vi "Multicard III_Hardware_Module.vi"(5 "Multicard (T:Enable)":bool=TRUE, 6 "Timeout(s)":dbl=5.0, 7 "Command":T1, 8 "error in (no error)":errorcluster, 10 "Input Value":dbl, 11 "VISA resource name":refnum<visa-resource-name>="COM4") -> (0 "error out":errorcluster, 1 "Timeout":bool, 2 "Output Value":dbl=5.0, 3 "String":string)   [LabVIEW 2013]
uses:
  Multicard III_Hardware_Module Control.ctl
  <vilib>/Instr/_visa.llb/VISA Configure Serial Port (Instr).vi
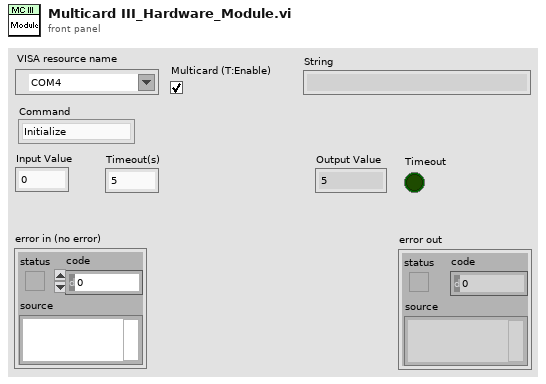
[diagram p1: front panel]
types:
  T1 = typedef "Multicard III_Hardware_Module Control.ctl" = enum16{"Initialize", "Cero", "Span", "Read ugr", "Read mgr", "Read A/D", "Read T", "Number readings", "Thermocouple type", "Status", "Shutdown"}
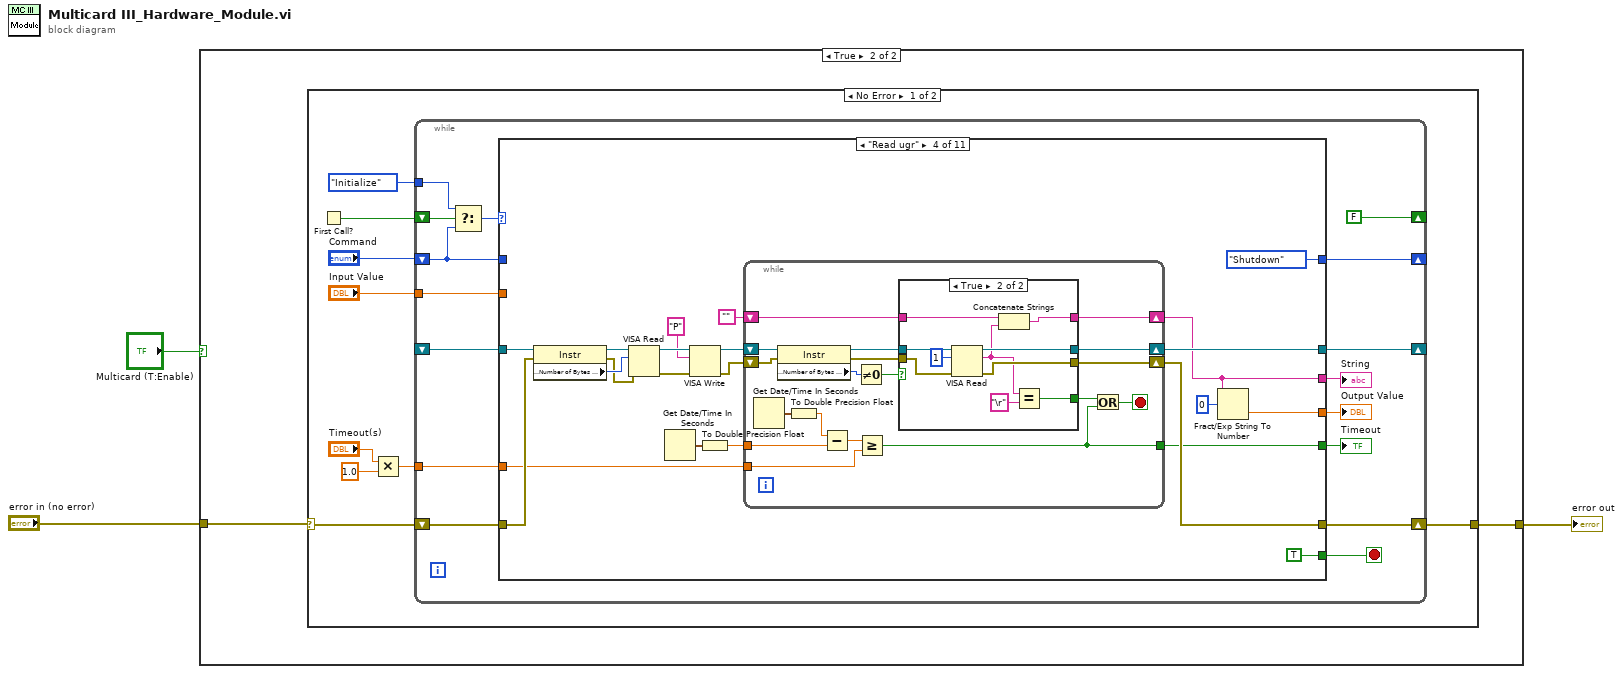
[diagram p0: block diagram]
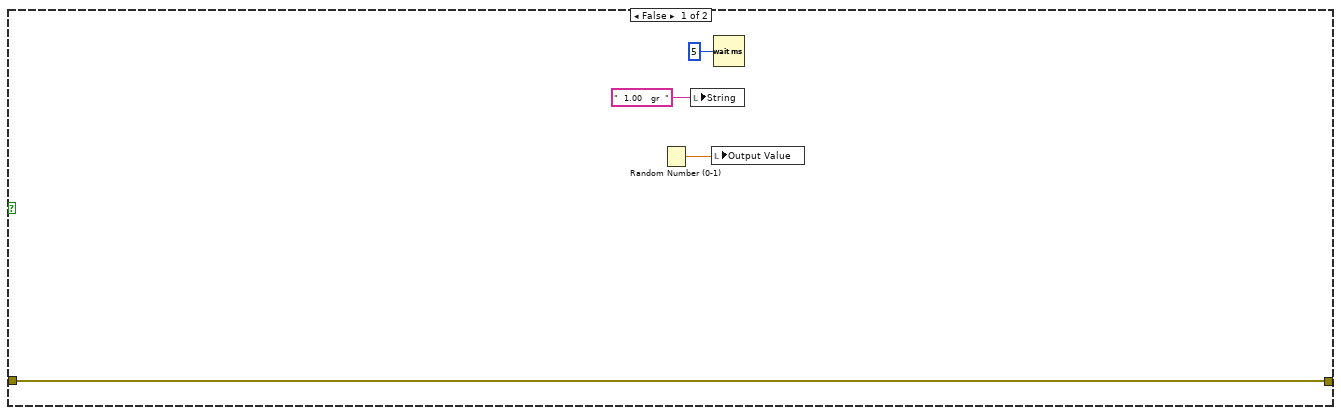
[diagram p2: hidden frame]
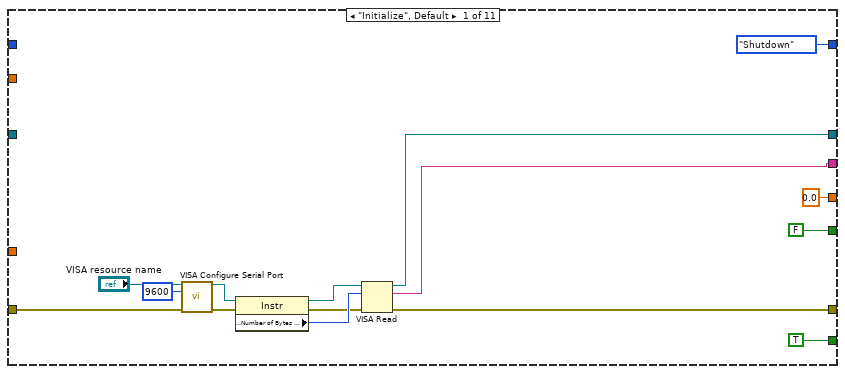
[diagram p3: hidden frame]
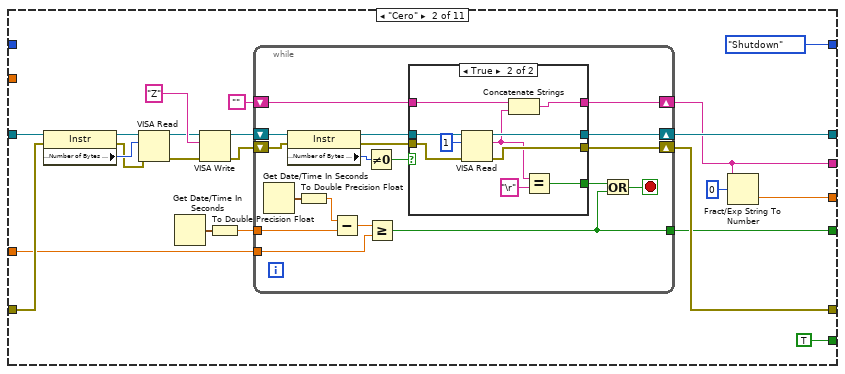
[diagram p4: hidden frame]
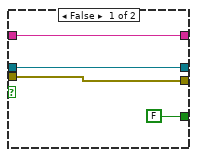
[diagram p5: hidden frame]
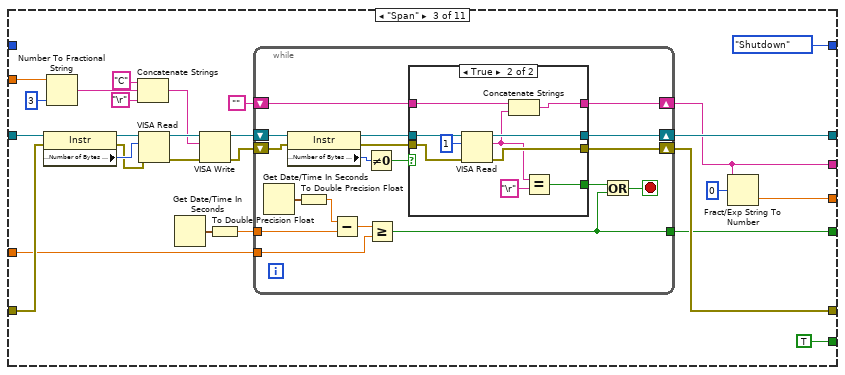
[diagram p6: hidden frame]
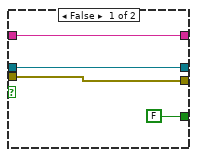
[diagram p7: hidden frame]
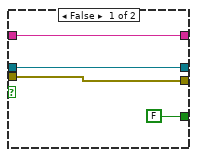
[diagram p8: hidden frame]
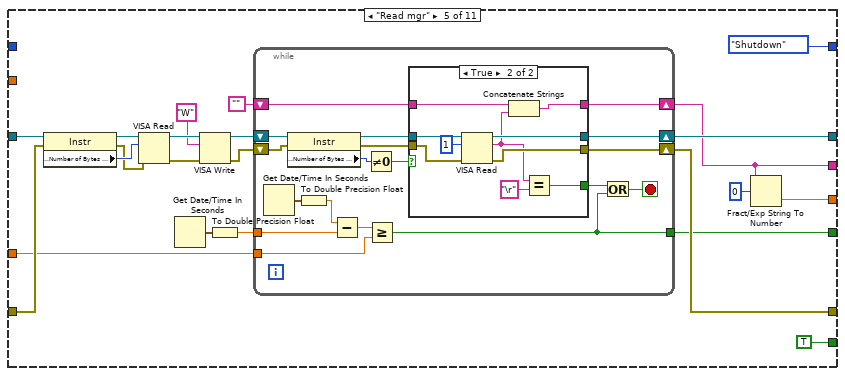
[diagram p9: hidden frame]
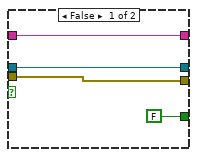
[diagram p10: hidden frame]
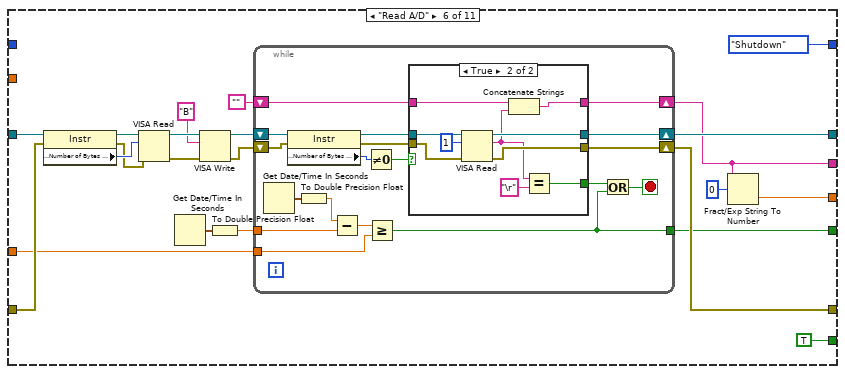
[diagram p11: hidden frame]
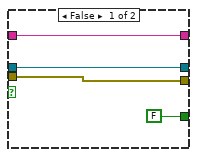
[diagram p12: hidden frame]
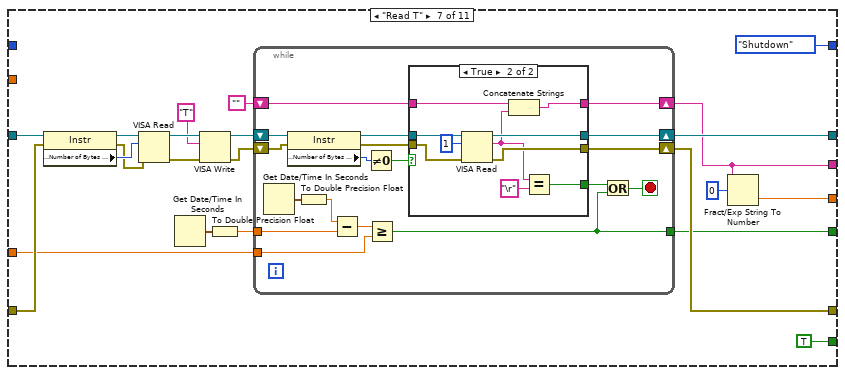
[diagram p13: hidden frame]
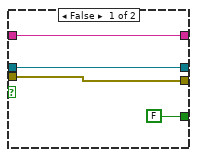
[diagram p14: hidden frame]
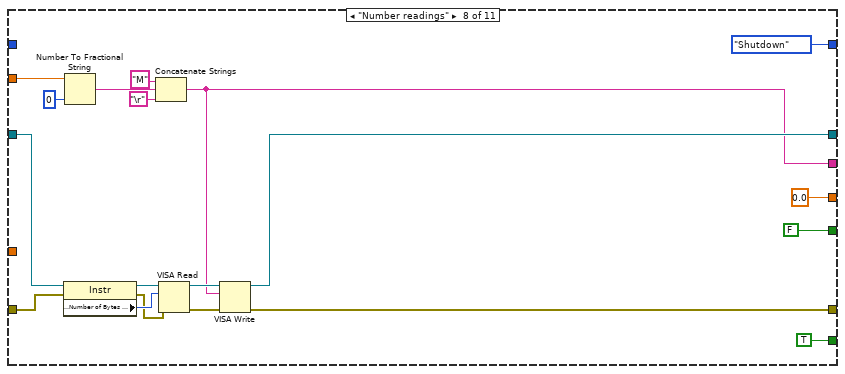
[diagram p15: hidden frame]
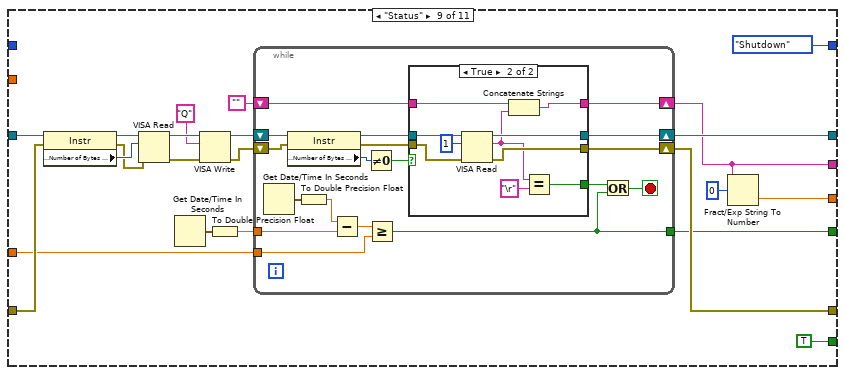
[diagram p16: hidden frame]
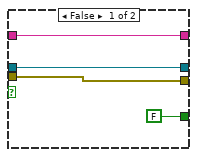
[diagram p17: hidden frame]
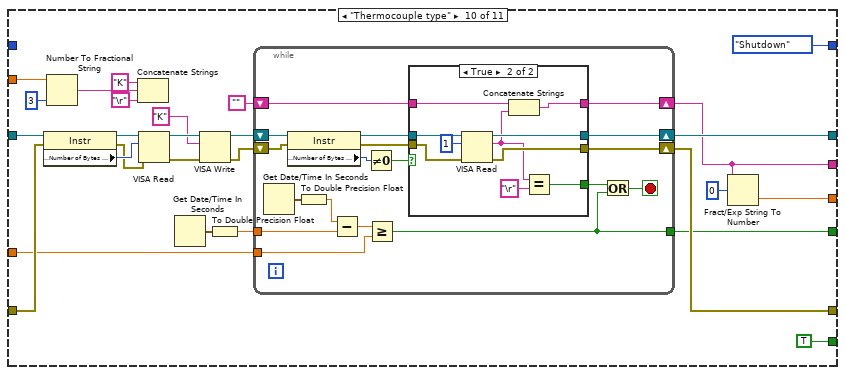
[diagram p18: hidden frame]
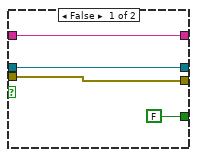
[diagram p19: hidden frame]
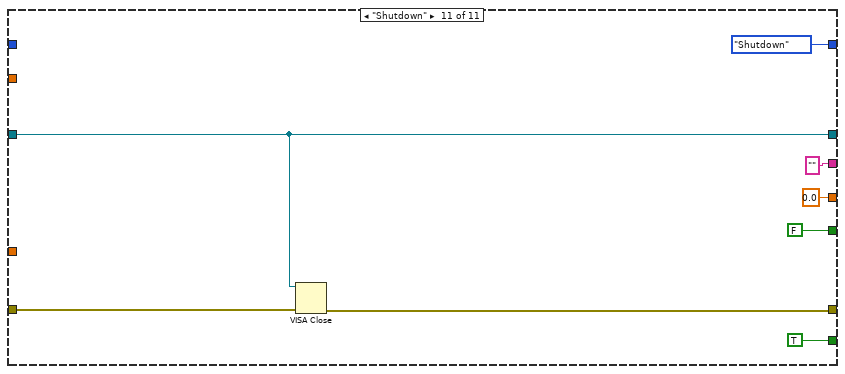
[diagram p20: hidden frame]
diagram:
  n1 = case shown="True" "Multicard (T:Enable)" {
    tunnel: "error in (no error)" -> [w7 w9]
    tunnel: [w7 w8] -> w2
    frame False {
      n2 = Random Number (0-1)() -> (number: 0 to 1=w5:dbl)
      n3 = local write "String"("  1.00   gr  " ("String")) -> ()
      n4 = local write "Output Value"(w5) -> ()
      n5 = Wait (ms)(milliseconds to wait=u32 5) -> ()  [unwired: 1 out]
    }
    frame True {
      n6 = case shown="No Error" w9 {
        selector: w9 -> [w16 w519]
        tunnel: [w15 w519] -> w8
        frame No Error {
          n7 = First Call?() -> (First Call?: T/F=w18:bool)
          n8 = Multiply(x="Timeout(s)", y=1.0) -> (x*y=w11:dbl)
          n9 = while {
            shift-right: [w26] -> _
            shift-left: "Command" -> [w27]
            shift-right: [w29] -> w15
            shift-left: w16 -> [w30]
            shift-right: [FALSE ("First Call?: T/F")] -> _
            shift-left: w18 -> [w34]
            tunnel: Multicard_III_Hardware_Module_Control."Initialize" ("t") -> [w33]
            shift-right: [w24] -> _
            shift-left: _ -> [w25]
            tunnel: w11 -> [w22]
            tunnel: "Input Value" -> [w19]
            stop <- w31 stop-if-true
            n10 = Select(t=w33, s=w34, f=w27) -> (s? t:f=w32:T1)
            n11 = case shown="\"Read ugr\"" w32 {
              tunnel: [TRUE TRUE TRUE TRUE TRUE TRUE TRUE TRUE TRUE TRUE TRUE] -> w31
              tunnel: w30 -> [w46 w58 w118 w172 w226 w280 w334 w390 w407 w466 w518]
              tunnel: [w39 w59 w119 w173 w227 w281 w335 w379 w408 w467 w517] -> w29
              tunnel: w27 -> [_ _ _ _ _ _ _ _ _ _ _]
              tunnel: [Multicard_III_Hardware_Module_Control."Shutdown" ("t") Multicard_III_Hardware_Module_Control."Shutdown" ("t") Multicard_III_Hardware_Module_Control."Shutdown" ("t") Multicard_III_Hardware_Module_Control."Shutdown" ("t") Multicard_III_Hardware_Module_Control."Shutdown" ("t") Multicard_III_Hardware_Module_Control."Shutdown" ("t") Multicard_III_Hardware_Module_Control."Shutdown" ("t") Multicard_III_Hardware_Module_Control."Shutdown" ("t") Multicard_III_Hardware_Module_Control."Shutdown" ("t") Multicard_III_Hardware_Module_Control."Shutdown" ("t") Multicard_III_Hardware_Module_Control."Shutdown" ("t")] -> w26
              tunnel: w25 -> [_ w57 w117 w171 w225 w279 w333 w389 w406 w465 w516]
              tunnel: [w38 w55 w115 w169 w223 w277 w331 w383 w404 w463 w516] -> w24
              tunnel: [w36 w52 w112 w166 w220 w274 w328 w382 w401 w460 ""] -> w23
              tunnel: w22 -> [_ w56 w116 w170 w224 w278 w332 _ w405 w464 _]
              tunnel: [FALSE w53 w113 w167 w221 w275 w329 FALSE w402 w461 FALSE] -> w21
              tunnel: [0.0 w51 w111 w165 w219 w273 w327 0.0 w400 w459 0.0] -> w20
              tunnel: w19 -> [_ _ w106 _ _ _ _ w384 _ w456 _]
              frame "Initialize", Default {
                n12 = call-poly "VISA Configure Serial Port"("VISA resource name"="VISA resource name", "baud rate (9600)"=u32 9600, "error in (no error)"=w46) -> ("VISA resource name out"=w41:refnum<visa-resource-name>, "error out"=w40:errorcluster)  [unwired: 11 in]
                n13 = property class="Instr"(reference=w41, error in=w40) -> (reference out=w42:refnum<visa-resource-name>, error out=w43:errorcluster, "Serial Settings:Number of Bytes at Serial Port"=w44:u32)
                n14 = VISA Read(VISA resource name=w42, byte count=w44, error in (no error)=w43) -> (VISA resource name out=w38:refnum<visa-resource-name>, read buffer=w36:string, error out=w39:errorcluster)  [unwired: 1 out]
              }
              frame "Cero" {
                n15 = property class="Instr"(reference=w57, error in=w58) -> (reference out=w66:refnum<visa-resource-name>, error out=w67:errorcluster, "Serial Settings:Number of Bytes at Serial Port"=w68:u32)
                n16 = VISA Read(VISA resource name=w66, byte count=w68, error in (no error)=w67) -> (VISA resource name out=w65:refnum<visa-resource-name>, error out=w64:errorcluster)  [unwired: 2 out]
                n17 = Get Date/Time In Seconds() -> (seconds since 1Jan1904=w63:timestamp)
                n18 = VISA Write(VISA resource name=w65, write buffer="Z" ("Mide"), error in (no error)=w64) -> (VISA resource name out=w61:refnum<visa-resource-name>, error out=w60:errorcluster)  [unwired: 1 out]
                n19 = To Double Precision Float(number=w63) -> (double precision float=w62:dbl)
                n20 = while {
                  tunnel: w62 -> [w86]
                  shift-right: [w82] -> w55
                  shift-left: w61 -> [w80]
                  shift-right: [w81] -> w59
                  shift-left: w60 -> [w79]
                  tunnel: w56 -> [w84]
                  tunnel: [w83] -> w53
                  shift-right: [w73] -> w52
                  shift-left: "" -> [w74]
                  stop <- w89 stop-if-true
                  n21 = Get Date/Time In Seconds() -> (seconds since 1Jan1904=w88:timestamp)
                  n22 = property class="Instr"(reference=w80, error in=w79) -> (reference out=w77:refnum<visa-resource-name>, error out=w78:errorcluster, "Serial Settings:Number of Bytes at Serial Port"=w76:u32)
                  n23 = To Double Precision Float(number=w88) -> (double precision float=w87:dbl)
                  n24 = Subtract(x=w87, y=w86) -> (x-y=w85:dbl)
                  n25 = Not Equal To 0?(x=w76) -> (x != 0?=w75:bool)
                  n26 = Greater Or Equal?(x=w85, y=w84) -> (x >= y?=w83:bool)
                  n27 = case shown="True" w75 {
                    tunnel: [w93 w103] -> w82
                    tunnel: [w92 w102] -> w81
                    tunnel: w78 -> [w92 w101]
                    tunnel: w77 -> [w93 w100]
                    tunnel: w74 -> [w91 w99]
                    tunnel: [w91 w98] -> w73
                    tunnel: [FALSE w94] -> w72
                    frame False {
                    }
                    frame True {
                      n28 = VISA Read(VISA resource name=w100, byte count=u32 1, error in (no error)=w101) -> (VISA resource name out=w103:refnum<visa-resource-name>, read buffer=w96:string, error out=w102:errorcluster)  [unwired: 1 out]
                      n29 = Concatenate Strings(w99, w96) -> (w98:string)
                      n30 = Equal?(x=w96, y="\r" ("Mide")) -> (x = y?=w94:bool)
                    }
                  }
                  n31 = Or(x=w72, y=w83) -> (x .or. y?=w89:bool)
                }
                n32 = Fract/Exp String To Number(string=w52, offset=0) -> (number=w51:dbl)  [unwired: 2 in, 1 out]
              }
              frame "Span" {
                n33 = property class="Instr"(reference=w117, error in=w118) -> (reference out=w126:refnum<visa-resource-name>, error out=w127:errorcluster, "Serial Settings:Number of Bytes at Serial Port"=w128:u32)
                n34 = Number To Fractional String(number=w106, precision (6)=i16 3) -> (F-format string=w104:string)  [unwired: 2 in]
                n35 = Concatenate Strings("C" ("Mide"), w104, "\r") -> (w107:string)
                n36 = VISA Read(VISA resource name=w126, byte count=w128, error in (no error)=w127) -> (VISA resource name out=w125:refnum<visa-resource-name>, error out=w124:errorcluster)  [unwired: 2 out]
                n37 = Get Date/Time In Seconds() -> (seconds since 1Jan1904=w123:timestamp)
                n38 = VISA Write(VISA resource name=w125, write buffer=w107, error in (no error)=w124) -> (VISA resource name out=w121:refnum<visa-resource-name>, error out=w120:errorcluster)  [unwired: 1 out]
                n39 = To Double Precision Float(number=w123) -> (double precision float=w122:dbl)
                n40 = while {
                  tunnel: w122 -> [w145]
                  shift-right: [w141] -> w115
                  shift-left: w121 -> [w139]
                  shift-right: [w140] -> w119
                  shift-left: w120 -> [w138]
                  tunnel: w116 -> [w143]
                  tunnel: [w142] -> w113
                  shift-right: [w132] -> w112
                  shift-left: "" -> [w133]
                  stop <- w148 stop-if-true
                  n41 = Get Date/Time In Seconds() -> (seconds since 1Jan1904=w147:timestamp)
                  n42 = property class="Instr"(reference=w139, error in=w138) -> (reference out=w136:refnum<visa-resource-name>, error out=w137:errorcluster, "Serial Settings:Number of Bytes at Serial Port"=w135:u32)
                  n43 = To Double Precision Float(number=w147) -> (double precision float=w146:dbl)
                  n44 = Subtract(x=w146, y=w145) -> (x-y=w144:dbl)
                  n45 = Not Equal To 0?(x=w135) -> (x != 0?=w134:bool)
                  n46 = Greater Or Equal?(x=w144, y=w143) -> (x >= y?=w142:bool)
                  n47 = case shown="True" w134 {
                    tunnel: [w152 w162] -> w141
                    tunnel: [w151 w161] -> w140
                    tunnel: w137 -> [w151 w160]
                    tunnel: w136 -> [w152 w159]
                    tunnel: w133 -> [w150 w158]
                    tunnel: [w150 w157] -> w132
                    tunnel: [FALSE w153] -> w131
                    frame False {
                    }
                    frame True {
                      n48 = VISA Read(VISA resource name=w159, byte count=u32 1, error in (no error)=w160) -> (VISA resource name out=w162:refnum<visa-resource-name>, read buffer=w155:string, error out=w161:errorcluster)  [unwired: 1 out]
                      n49 = Concatenate Strings(w158, w155) -> (w157:string)
                      n50 = Equal?(x=w155, y="\r" ("Mide")) -> (x = y?=w153:bool)
                    }
                  }
                  n51 = Or(x=w131, y=w142) -> (x .or. y?=w148:bool)
                }
                n52 = Fract/Exp String To Number(string=w112, offset=0) -> (number=w111:dbl)  [unwired: 2 in, 1 out]
              }
              frame "Read ugr" {
                n53 = property class="Instr"(reference=w171, error in=w172) -> (reference out=w180:refnum<visa-resource-name>, error out=w181:errorcluster, "Serial Settings:Number of Bytes at Serial Port"=w182:u32)
                n54 = VISA Read(VISA resource name=w180, byte count=w182, error in (no error)=w181) -> (VISA resource name out=w179:refnum<visa-resource-name>, error out=w178:errorcluster)  [unwired: 2 out]
                n55 = Get Date/Time In Seconds() -> (seconds since 1Jan1904=w177:timestamp)
                n56 = VISA Write(VISA resource name=w179, write buffer="P", error in (no error)=w178) -> (VISA resource name out=w175:refnum<visa-resource-name>, error out=w174:errorcluster)  [unwired: 1 out]
                n57 = To Double Precision Float(number=w177) -> (double precision float=w176:dbl)
                n58 = while {
                  tunnel: w176 -> [w199]
                  shift-right: [w195] -> w169
                  shift-left: w175 -> [w193]
                  shift-right: [w194] -> w173
                  shift-left: w174 -> [w192]
                  tunnel: w170 -> [w197]
                  tunnel: [w196] -> w167
                  shift-right: [w186] -> w166
                  shift-left: "" -> [w187]
                  stop <- w202 stop-if-true
                  n59 = Get Date/Time In Seconds() -> (seconds since 1Jan1904=w201:timestamp)
                  n60 = property class="Instr"(reference=w193, error in=w192) -> (reference out=w190:refnum<visa-resource-name>, error out=w191:errorcluster, "Serial Settings:Number of Bytes at Serial Port"=w189:u32)
                  n61 = To Double Precision Float(number=w201) -> (double precision float=w200:dbl)
                  n62 = Subtract(x=w200, y=w199) -> (x-y=w198:dbl)
                  n63 = Not Equal To 0?(x=w189) -> (x != 0?=w188:bool)
                  n64 = Greater Or Equal?(x=w198, y=w197) -> (x >= y?=w196:bool)
                  n65 = case shown="True" w188 {
                    tunnel: [w206 w216] -> w195
                    tunnel: [w205 w215] -> w194
                    tunnel: w191 -> [w205 w214]
                    tunnel: w190 -> [w206 w213]
                    tunnel: w187 -> [w204 w212]
                    tunnel: [w204 w211] -> w186
                    tunnel: [FALSE w207] -> w185
                    frame False {
                    }
                    frame True {
                      n66 = VISA Read(VISA resource name=w213, byte count=u32 1, error in (no error)=w214) -> (VISA resource name out=w216:refnum<visa-resource-name>, read buffer=w209:string, error out=w215:errorcluster)  [unwired: 1 out]
                      n67 = Concatenate Strings(w212, w209) -> (w211:string)
                      n68 = Equal?(x=w209, y="\r" ("Mide")) -> (x = y?=w207:bool)
                    }
                  }
                  n69 = Or(x=w185, y=w196) -> (x .or. y?=w202:bool)
                }
                n70 = Fract/Exp String To Number(string=w166, offset=0) -> (number=w165:dbl)  [unwired: 2 in, 1 out]
              }
              frame "Read mgr" {
                n71 = property class="Instr"(reference=w225, error in=w226) -> (reference out=w234:refnum<visa-resource-name>, error out=w235:errorcluster, "Serial Settings:Number of Bytes at Serial Port"=w236:u32)
                n72 = VISA Read(VISA resource name=w234, byte count=w236, error in (no error)=w235) -> (VISA resource name out=w233:refnum<visa-resource-name>, error out=w232:errorcluster)  [unwired: 2 out]
                n73 = Get Date/Time In Seconds() -> (seconds since 1Jan1904=w231:timestamp)
                n74 = VISA Write(VISA resource name=w233, write buffer="W" ("Mide"), error in (no error)=w232) -> (VISA resource name out=w229:refnum<visa-resource-name>, error out=w228:errorcluster)  [unwired: 1 out]
                n75 = To Double Precision Float(number=w231) -> (double precision float=w230:dbl)
                n76 = while {
                  tunnel: w230 -> [w253]
                  shift-right: [w249] -> w223
                  shift-left: w229 -> [w247]
                  shift-right: [w248] -> w227
                  shift-left: w228 -> [w246]
                  tunnel: w224 -> [w251]
                  tunnel: [w250] -> w221
                  shift-right: [w240] -> w220
                  shift-left: "" -> [w241]
                  stop <- w256 stop-if-true
                  n77 = Get Date/Time In Seconds() -> (seconds since 1Jan1904=w255:timestamp)
                  n78 = property class="Instr"(reference=w247, error in=w246) -> (reference out=w244:refnum<visa-resource-name>, error out=w245:errorcluster, "Serial Settings:Number of Bytes at Serial Port"=w243:u32)
                  n79 = To Double Precision Float(number=w255) -> (double precision float=w254:dbl)
                  n80 = Subtract(x=w254, y=w253) -> (x-y=w252:dbl)
                  n81 = Not Equal To 0?(x=w243) -> (x != 0?=w242:bool)
                  n82 = Greater Or Equal?(x=w252, y=w251) -> (x >= y?=w250:bool)
                  n83 = case shown="True" w242 {
                    tunnel: [w260 w270] -> w249
                    tunnel: [w259 w269] -> w248
                    tunnel: w245 -> [w259 w268]
                    tunnel: w244 -> [w260 w267]
                    tunnel: w241 -> [w258 w266]
                    tunnel: [w258 w265] -> w240
                    tunnel: [FALSE w261] -> w239
                    frame False {
                    }
                    frame True {
                      n84 = VISA Read(VISA resource name=w267, byte count=u32 1, error in (no error)=w268) -> (VISA resource name out=w270:refnum<visa-resource-name>, read buffer=w263:string, error out=w269:errorcluster)  [unwired: 1 out]
                      n85 = Concatenate Strings(w266, w263) -> (w265:string)
                      n86 = Equal?(x=w263, y="\r" ("Mide")) -> (x = y?=w261:bool)
                    }
                  }
                  n87 = Or(x=w239, y=w250) -> (x .or. y?=w256:bool)
                }
                n88 = Fract/Exp String To Number(string=w220, offset=0) -> (number=w219:dbl)  [unwired: 2 in, 1 out]
              }
              frame "Read A/D" {
                n89 = property class="Instr"(reference=w279, error in=w280) -> (reference out=w288:refnum<visa-resource-name>, error out=w289:errorcluster, "Serial Settings:Number of Bytes at Serial Port"=w290:u32)
                n90 = VISA Read(VISA resource name=w288, byte count=w290, error in (no error)=w289) -> (VISA resource name out=w287:refnum<visa-resource-name>, error out=w286:errorcluster)  [unwired: 2 out]
                n91 = Get Date/Time In Seconds() -> (seconds since 1Jan1904=w285:timestamp)
                n92 = VISA Write(VISA resource name=w287, write buffer="B", error in (no error)=w286) -> (VISA resource name out=w283:refnum<visa-resource-name>, error out=w282:errorcluster)  [unwired: 1 out]
                n93 = To Double Precision Float(number=w285) -> (double precision float=w284:dbl)
                n94 = while {
                  tunnel: w284 -> [w307]
                  shift-right: [w303] -> w277
                  shift-left: w283 -> [w301]
                  shift-right: [w302] -> w281
                  shift-left: w282 -> [w300]
                  tunnel: w278 -> [w305]
                  tunnel: [w304] -> w275
                  shift-right: [w294] -> w274
                  shift-left: "" -> [w295]
                  stop <- w310 stop-if-true
                  n95 = Get Date/Time In Seconds() -> (seconds since 1Jan1904=w309:timestamp)
                  n96 = property class="Instr"(reference=w301, error in=w300) -> (reference out=w298:refnum<visa-resource-name>, error out=w299:errorcluster, "Serial Settings:Number of Bytes at Serial Port"=w297:u32)
                  n97 = To Double Precision Float(number=w309) -> (double precision float=w308:dbl)
                  n98 = Subtract(x=w308, y=w307) -> (x-y=w306:dbl)
                  n99 = Not Equal To 0?(x=w297) -> (x != 0?=w296:bool)
                  n100 = Greater Or Equal?(x=w306, y=w305) -> (x >= y?=w304:bool)
                  n101 = case shown="True" w296 {
                    tunnel: [w314 w324] -> w303
                    tunnel: [w313 w323] -> w302
                    tunnel: w299 -> [w313 w322]
                    tunnel: w298 -> [w314 w321]
                    tunnel: w295 -> [w312 w320]
                    tunnel: [w312 w319] -> w294
                    tunnel: [FALSE w315] -> w293
                    frame False {
                    }
                    frame True {
                      n102 = VISA Read(VISA resource name=w321, byte count=u32 1, error in (no error)=w322) -> (VISA resource name out=w324:refnum<visa-resource-name>, read buffer=w317:string, error out=w323:errorcluster)  [unwired: 1 out]
                      n103 = Concatenate Strings(w320, w317) -> (w319:string)
                      n104 = Equal?(x=w317, y="\r" ("Mide")) -> (x = y?=w315:bool)
                    }
                  }
                  n105 = Or(x=w293, y=w304) -> (x .or. y?=w310:bool)
                }
                n106 = Fract/Exp String To Number(string=w274, offset=0) -> (number=w273:dbl)  [unwired: 2 in, 1 out]
              }
              frame "Read T" {
                n107 = property class="Instr"(reference=w333, error in=w334) -> (reference out=w342:refnum<visa-resource-name>, error out=w343:errorcluster, "Serial Settings:Number of Bytes at Serial Port"=w344:u32)
                n108 = VISA Read(VISA resource name=w342, byte count=w344, error in (no error)=w343) -> (VISA resource name out=w341:refnum<visa-resource-name>, error out=w340:errorcluster)  [unwired: 2 out]
                n109 = Get Date/Time In Seconds() -> (seconds since 1Jan1904=w339:timestamp)
                n110 = VISA Write(VISA resource name=w341, write buffer="T", error in (no error)=w340) -> (VISA resource name out=w337:refnum<visa-resource-name>, error out=w336:errorcluster)  [unwired: 1 out]
                n111 = To Double Precision Float(number=w339) -> (double precision float=w338:dbl)
                n112 = while {
                  tunnel: w338 -> [w361]
                  shift-right: [w357] -> w331
                  shift-left: w337 -> [w355]
                  shift-right: [w356] -> w335
                  shift-left: w336 -> [w354]
                  tunnel: w332 -> [w359]
                  tunnel: [w358] -> w329
                  shift-right: [w348] -> w328
                  shift-left: "" -> [w349]
                  stop <- w364 stop-if-true
                  n113 = Get Date/Time In Seconds() -> (seconds since 1Jan1904=w363:timestamp)
                  n114 = property class="Instr"(reference=w355, error in=w354) -> (reference out=w352:refnum<visa-resource-name>, error out=w353:errorcluster, "Serial Settings:Number of Bytes at Serial Port"=w351:u32)
                  n115 = To Double Precision Float(number=w363) -> (double precision float=w362:dbl)
                  n116 = Subtract(x=w362, y=w361) -> (x-y=w360:dbl)
                  n117 = Not Equal To 0?(x=w351) -> (x != 0?=w350:bool)
                  n118 = Greater Or Equal?(x=w360, y=w359) -> (x >= y?=w358:bool)
                  n119 = case shown="True" w350 {
                    tunnel: [w368 w378] -> w357
                    tunnel: [w367 w377] -> w356
                    tunnel: w353 -> [w367 w376]
                    tunnel: w352 -> [w368 w375]
                    tunnel: w349 -> [w366 w374]
                    tunnel: [w366 w373] -> w348
                    tunnel: [FALSE w369] -> w347
                    frame False {
                    }
                    frame True {
                      n120 = VISA Read(VISA resource name=w375, byte count=u32 1, error in (no error)=w376) -> (VISA resource name out=w378:refnum<visa-resource-name>, read buffer=w371:string, error out=w377:errorcluster)  [unwired: 1 out]
                      n121 = Concatenate Strings(w374, w371) -> (w373:string)
                      n122 = Equal?(x=w371, y="\r" ("Mide")) -> (x = y?=w369:bool)
                    }
                  }
                  n123 = Or(x=w347, y=w358) -> (x .or. y?=w364:bool)
                }
                n124 = Fract/Exp String To Number(string=w328, offset=0) -> (number=w327:dbl)  [unwired: 2 in, 1 out]
              }
              frame "Number readings" {
                n125 = property class="Instr"(reference=w389, error in=w390) -> (reference out=w393:refnum<visa-resource-name>, error out=w394:errorcluster, "Serial Settings:Number of Bytes at Serial Port"=w395:u32)
                n126 = Number To Fractional String(number=w384, precision (6)=i16 0) -> (F-format string=w385:string)  [unwired: 2 in]
                n127 = Concatenate Strings("M" ("Mide"), w385, "\r") -> (w382:string)
                n128 = VISA Read(VISA resource name=w393, byte count=w395, error in (no error)=w394) -> (VISA resource name out=w392:refnum<visa-resource-name>, error out=w391:errorcluster)  [unwired: 2 out]
                n129 = VISA Write(VISA resource name=w392, write buffer=w382, error in (no error)=w391) -> (VISA resource name out=w383:refnum<visa-resource-name>, error out=w379:errorcluster)  [unwired: 1 out]
              }
              frame "Status" {
                n130 = property class="Instr"(reference=w406, error in=w407) -> (reference out=w415:refnum<visa-resource-name>, error out=w416:errorcluster, "Serial Settings:Number of Bytes at Serial Port"=w417:u32)
                n131 = VISA Read(VISA resource name=w415, byte count=w417, error in (no error)=w416) -> (VISA resource name out=w414:refnum<visa-resource-name>, error out=w413:errorcluster)  [unwired: 2 out]
                n132 = Get Date/Time In Seconds() -> (seconds since 1Jan1904=w412:timestamp)
                n133 = VISA Write(VISA resource name=w414, write buffer="Q" ("Mide"), error in (no error)=w413) -> (VISA resource name out=w410:refnum<visa-resource-name>, error out=w409:errorcluster)  [unwired: 1 out]
                n134 = To Double Precision Float(number=w412) -> (double precision float=w411:dbl)
                n135 = while {
                  tunnel: w411 -> [w434]
                  shift-right: [w430] -> w404
                  shift-left: w410 -> [w428]
                  shift-right: [w429] -> w408
                  shift-left: w409 -> [w427]
                  tunnel: w405 -> [w432]
                  tunnel: [w431] -> w402
                  shift-right: [w421] -> w401
                  shift-left: "" -> [w422]
                  stop <- w437 stop-if-true
                  n136 = Get Date/Time In Seconds() -> (seconds since 1Jan1904=w436:timestamp)
                  n137 = property class="Instr"(reference=w428, error in=w427) -> (reference out=w425:refnum<visa-resource-name>, error out=w426:errorcluster, "Serial Settings:Number of Bytes at Serial Port"=w424:u32)
                  n138 = To Double Precision Float(number=w436) -> (double precision float=w435:dbl)
                  n139 = Subtract(x=w435, y=w434) -> (x-y=w433:dbl)
                  n140 = Not Equal To 0?(x=w424) -> (x != 0?=w423:bool)
                  n141 = Greater Or Equal?(x=w433, y=w432) -> (x >= y?=w431:bool)
                  n142 = case shown="True" w423 {
                    tunnel: [w441 w451] -> w430
                    tunnel: [w440 w450] -> w429
                    tunnel: w426 -> [w440 w449]
                    tunnel: w425 -> [w441 w448]
                    tunnel: w422 -> [w439 w447]
                    tunnel: [w439 w446] -> w421
                    tunnel: [FALSE w442] -> w420
                    frame False {
                    }
                    frame True {
                      n143 = VISA Read(VISA resource name=w448, byte count=u32 1, error in (no error)=w449) -> (VISA resource name out=w451:refnum<visa-resource-name>, read buffer=w444:string, error out=w450:errorcluster)  [unwired: 1 out]
                      n144 = Concatenate Strings(w447, w444) -> (w446:string)
                      n145 = Equal?(x=w444, y="\r" ("Mide")) -> (x = y?=w442:bool)
                    }
                  }
                  n146 = Or(x=w420, y=w431) -> (x .or. y?=w437:bool)
                }
                n147 = Fract/Exp String To Number(string=w401, offset=0) -> (number=w400:dbl)  [unwired: 2 in, 1 out]
              }
              frame "Thermocouple type" {
                n148 = property class="Instr"(reference=w465, error in=w466) -> (reference out=w474:refnum<visa-resource-name>, error out=w475:errorcluster, "Serial Settings:Number of Bytes at Serial Port"=w476:u32)
                n149 = Number To Fractional String(number=w456, precision (6)=i16 3) -> (F-format string=w454:string)  [unwired: 2 in]
                n150 = Concatenate Strings("K" ("string"), w454, "\r") -> ()  [unwired: 1 out]
                n151 = VISA Read(VISA resource name=w474, byte count=w476, error in (no error)=w475) -> (VISA resource name out=w473:refnum<visa-resource-name>, error out=w472:errorcluster)  [unwired: 2 out]
                n152 = Get Date/Time In Seconds() -> (seconds since 1Jan1904=w471:timestamp)
                n153 = VISA Write(VISA resource name=w473, write buffer="K" ("Mide"), error in (no error)=w472) -> (VISA resource name out=w469:refnum<visa-resource-name>, error out=w468:errorcluster)  [unwired: 1 out]
                n154 = To Double Precision Float(number=w471) -> (double precision float=w470:dbl)
                n155 = while {
                  tunnel: w470 -> [w493]
                  shift-right: [w489] -> w463
                  shift-left: w469 -> [w487]
                  shift-right: [w488] -> w467
                  shift-left: w468 -> [w486]
                  tunnel: w464 -> [w491]
                  tunnel: [w490] -> w461
                  shift-right: [w480] -> w460
                  shift-left: "" -> [w481]
                  stop <- w496 stop-if-true
                  n156 = Get Date/Time In Seconds() -> (seconds since 1Jan1904=w495:timestamp)
                  n157 = property class="Instr"(reference=w487, error in=w486) -> (reference out=w484:refnum<visa-resource-name>, error out=w485:errorcluster, "Serial Settings:Number of Bytes at Serial Port"=w483:u32)
                  n158 = To Double Precision Float(number=w495) -> (double precision float=w494:dbl)
                  n159 = Subtract(x=w494, y=w493) -> (x-y=w492:dbl)
                  n160 = Not Equal To 0?(x=w483) -> (x != 0?=w482:bool)
                  n161 = Greater Or Equal?(x=w492, y=w491) -> (x >= y?=w490:bool)
                  n162 = case shown="True" w482 {
                    tunnel: [w500 w510] -> w489
                    tunnel: [w499 w509] -> w488
                    tunnel: w485 -> [w499 w508]
                    tunnel: w484 -> [w500 w507]
                    tunnel: w481 -> [w498 w506]
                    tunnel: [w498 w505] -> w480
                    tunnel: [FALSE w501] -> w479
                    frame False {
                    }
                    frame True {
                      n163 = VISA Read(VISA resource name=w507, byte count=u32 1, error in (no error)=w508) -> (VISA resource name out=w510:refnum<visa-resource-name>, read buffer=w503:string, error out=w509:errorcluster)  [unwired: 1 out]
                      n164 = Concatenate Strings(w506, w503) -> (w505:string)
                      n165 = Equal?(x=w503, y="\r" ("Mide")) -> (x = y?=w501:bool)
                    }
                  }
                  n166 = Or(x=w479, y=w490) -> (x .or. y?=w496:bool)
                }
                n167 = Fract/Exp String To Number(string=w460, offset=0) -> (number=w459:dbl)  [unwired: 2 in, 1 out]
              }
              frame "Shutdown" {
                n168 = VISA Close(VISA resource name=w516, error in (no error)=w518) -> (error out=w517:errorcluster)
              }
            }
            "String" <- w23
            "Timeout" <- w21
            "Output Value" <- w20
          }
        }
        frame Error {
        }
      }
    }
  }
  "error out" <- w2
